vi "Webcam.vi"(7 "error in":errorcluster) -> (0 "error out":errorcluster, 1 "Frame Rate":dbl)   [LabVIEW 2018]
panel:
  in  "Max Radius (Circle Detection 1)":sgl=25.0
  in  "Min Radius (Circle Detection 1)":sgl=21.0
  out "original Image":T1(plugin-control)
  out "Ball Found":bool
  out "balls":i32
  out "Raw Circle Data":T2(array[cluster])
  out "Binary Image":T1(plugin-control)
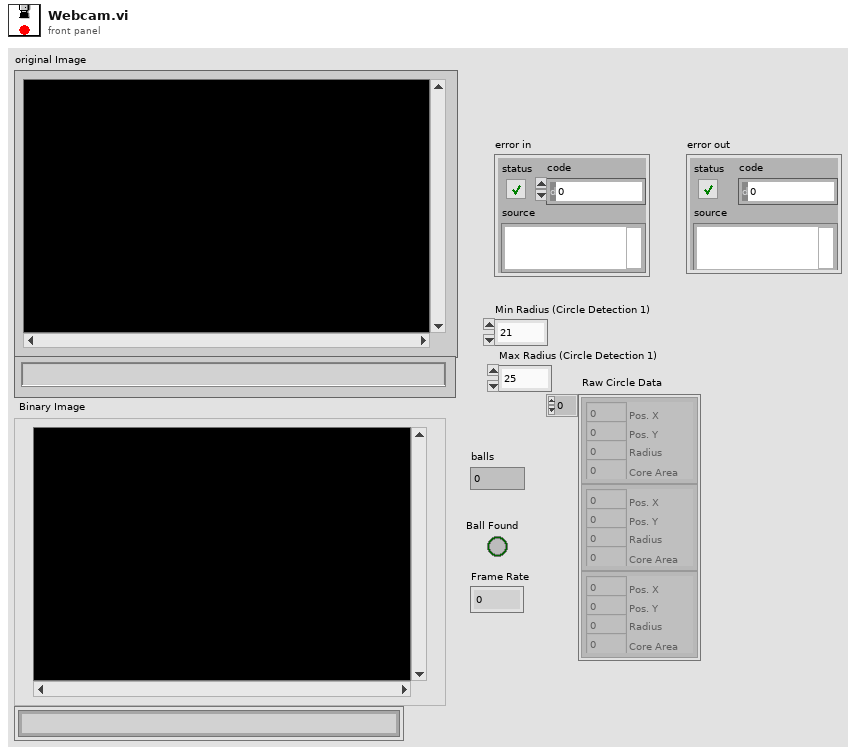
[diagram p1: front panel]
types:
  T1 = typedef "IMAQ Image.ctl" = refnum<image>
  T2 = cluster{"Pos. X":i32, "Pos. Y":i32, "Radius":i32, "Core Area":i32}[]
  T3 = cluster{"Pos. X":i32, "Pos. Y":i32, "Radius":i32, "Core Area":i32}
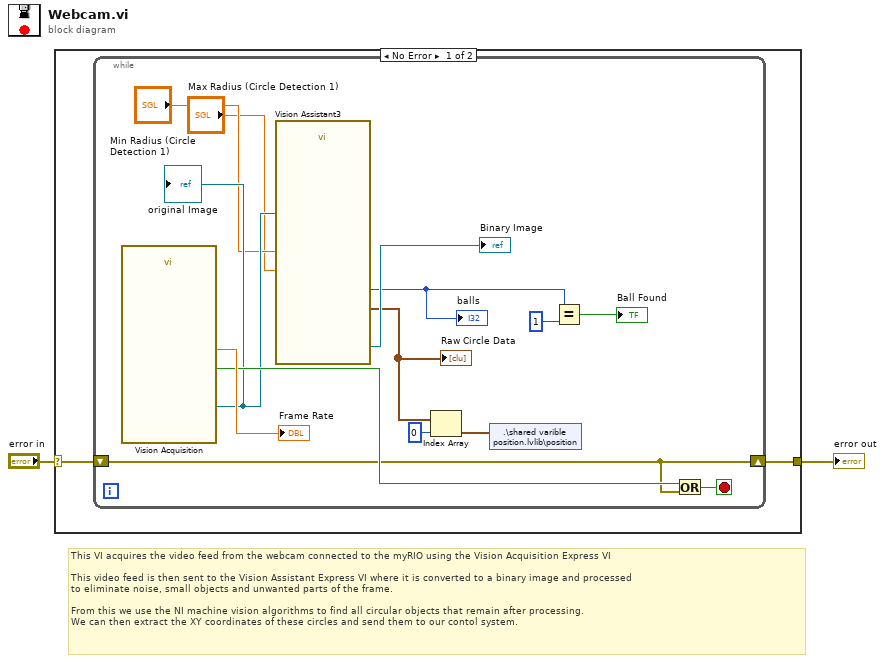
[diagram p0: block diagram]
diagram:
  # "This VI acquires the video feed from the webcam connected to the myRIO using the Vision Acquisition Express VI\n\nThis video feed is then sent to the Vision Assistant Express VI where it is converted to a binary image and processed\nto eliminate noise, small objects and unwanted parts of the frame.\n\nFrom this we use the NI machine vision algorithms to find all circular objects that remain after processing. \nWe can then extract the XY coordinates of these circles and send them to our contol system."
  n1 = case shown="No Error" "error in" {
    selector: "error in" -> [w3 w19]
    tunnel: [w4 w19] -> w2
    frame No Error {
      n2 = while {
        shift-right: [w7] -> w4
        shift-left: w3 -> [w7]
        stop <- w16 stop-if-true
        n3 = call "Vision Acquisition"() -> ("Image Out"=w10:T1, "Frame Rate"=→"Frame Rate":dbl, "Stopped"=w17:bool)  [unwired: 24 in, 1 out]
        "original Image" <- w10
        n4 = call "Vision Assistant3"("Image In"=w10, "Min Radius (Circle Detection 1)"="Min Radius (Circle Detection 1)", "Max Radius (Circle Detection 1)"="Max Radius (Circle Detection 1)") -> ("Image Out"=→"Binary Image":T1, "Nb Circles (Circle Detection 1)"=w13:i32, "Circles Data (Circle Detection 1)"=w14:T2)  [unwired: 20 in, 2 out]
        "Raw Circle Data" <- w14
        "balls" <- w13
        n5 = Index Array(array=w14, index=0) -> (element=w8:T3)
        n6 = shared-variable ".\\shared varible position.lvlib\\position"(w8) -> ()  [unwired: 1 in, 1 out]
        n7 = Equal?(x=w13, y=1) -> (x = y?=→"Ball Found":bool)
        n8 = Or(x=w17, y=w7) -> (x .or. y?=w16:bool)
      }
    }
    frame Error {
    }
  }
  "error out" <- w2
